vi "image to image.vi"() -> ()   [LabVIEW 2018]
uses:
  <vilib>/vision/Image Controls.llb/IMAQ Image.ctl
  <vilib>/vision/NI_Vision_Development_Module.lvlib
panel:
  out "Image Dst Out":T1
  out "error out":errorcluster
  in  "路径":path
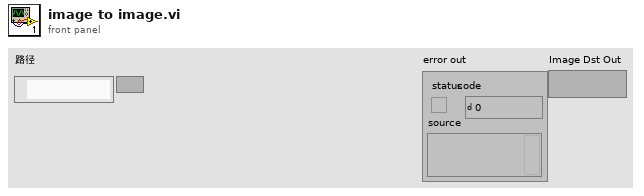
[diagram p1: front panel]
types:
  T1 = typedef "IMAQ Image.ctl" = refnum<image>
  T2 = typedef "Image Type" = u32
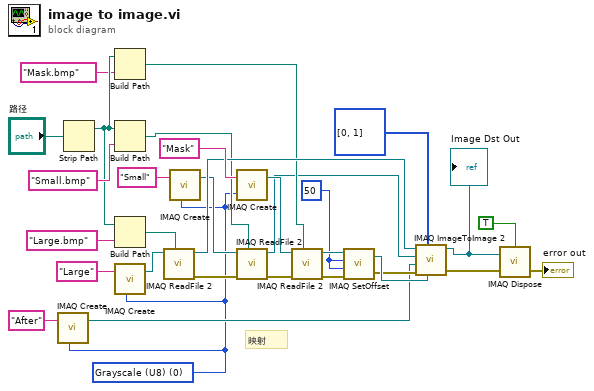
[diagram p0: block diagram]
diagram:
  w5 = T2 0 items=["Grayscale (U8)", "Grayscale (I16)", "Grayscale (SGL)", "Complex (CSG)", "RGB (U32)", "HSL (U32)", "RGB (U64)", "Grayscale (U16)"] ("Image Type")
  w9 = 50 ("X Offset")
  # "映射"
  n1 = call "IMAQ Create"("Image Name"="After", "Image Type"=w5) -> ("New Image"=w6:T1)  [unwired: 3 in, 1 out]
  n2 = Strip Path(path="路径") -> (stripped path=w19:path)  [unwired: 1 out]
  n3 = Build Path(base path=w19, name or relative path="Mask.bmp" ("名称或相对路径")) -> (appended path=w16:path)
  n4 = Build Path(base path=w19, name or relative path="Small.bmp" ("名称或相对路径")) -> (appended path=w20:path)
  n5 = Build Path(base path=w19, name or relative path="Large.bmp" ("名称或相对路径")) -> (appended path=w25:path)
  n6 = call "IMAQ Create"("Image Name"="Large", "Image Type"=w5) -> ("New Image"=w24:T1)  [unwired: 3 in, 1 out]
  n7 = call "IMAQ ReadFile 2"("File Path"=w25, "Image"=w24) -> ("error out"=w15:errorcluster, "Image Out"=w23:T1)  [unwired: 5 in, 3 out]
  n8 = call "IMAQ Create"("Image Name"="Small", "Image Type"=w5) -> ("New Image"=w21:T1)  [unwired: 3 in, 1 out]
  n9 = call "IMAQ Create"("Image Name"="Mask", "Image Type"=w5) -> ("New Image"=w17:T1)  [unwired: 3 in, 1 out]
  n10 = call "IMAQ ReadFile 2"("File Path"=w20, "error in (no error)"=w15, "Image"=w21) -> ("error out"=w14:errorcluster, "Image Out"=w13:T1)  [unwired: 4 in, 3 out]
  n11 = call "IMAQ ReadFile 2"("File Path"=w16, "error in (no error)"=w14, "Image"=w17) -> ("error out"=w10:errorcluster, "Image Out"=w11:T1)  [unwired: 4 in, 3 out]
  n12 = call "IMAQ SetOffset"("error in (no error)"=w10, "Y Offset"=w9, "X Offset"=w9, "Image"=w11) -> ("error out"=w7:errorcluster, "Image Out"=w8:T1)
  n13 = call "IMAQ ImageToImage 2"("Image Mask"=w8, "Offset Left/Top"=i32[] [0, 1], "error in (no error)"=w7, "Image Dst"=w6, "Image Src (Small)"=w13, "Image Src (Large)"=w23) -> ("error out"=w3:errorcluster, "Image Dst Out"=w4:T1)  [unwired: 4 in]
  "Image Dst Out" <- w4
  n14 = call "IMAQ Dispose"("All Images? (No)"=TRUE, "Image"=w4, "error in (no error)"=w3) -> ("error out"=→"error out":errorcluster)  [unwired: 3 in]
